vi "Get Bus.vi"(8 "error in (no error)":errorcluster, 11 "Local Bus_Int in":refnum<class "Local Bus_Int.lvclass">) -> (0 "error out":errorcluster, 2 "Bus":refnum<class "Local Bus.lvclass">, 3 "Local Bus_Int out":refnum<class "Local Bus_Int.lvclass">)   [LabVIEW 2021, in "Local Bus_Int.lvclass"]
uses:
  Local Bus_Int.lvclass
  Local Bus.lvclass
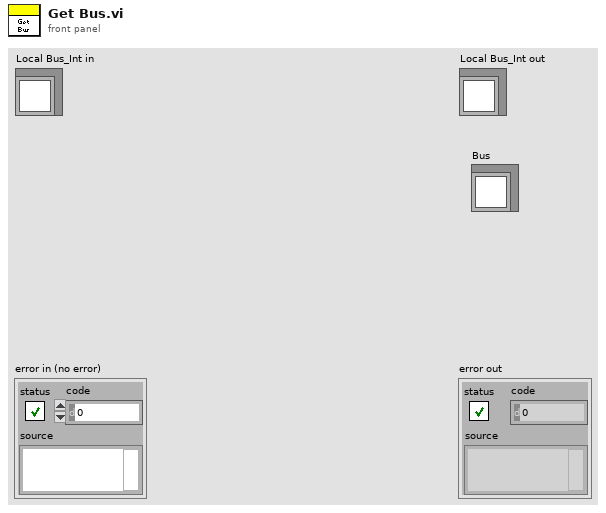
[diagram p1: front panel]
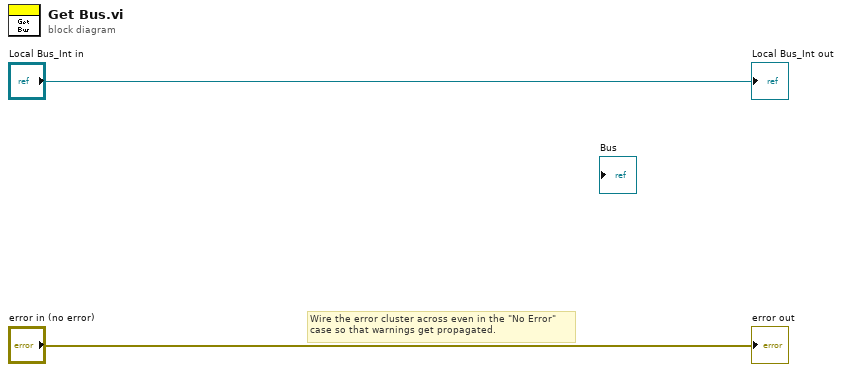
[diagram p0: block diagram]
diagram:
  # "Wire the error cluster across even in the \"No Error\"\ncase so that warnings get propagated."
  "error out" <- "error in (no error)"
  "Local Bus_Int out" <- "Local Bus_Int in"
